vi "WhatDoNow.vi"(10 "Target":dbl(slide) scale=-3.14159..3.14159, 11 "Current":dbl(slide) scale=-3.14159..3.14159) -> (2 "Invert":bool, 3 "Output":dbl)   [LabVIEW 2013]
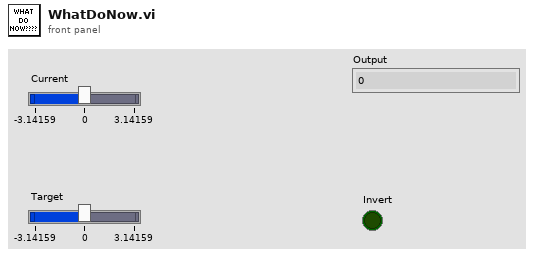
[diagram p1: front panel]
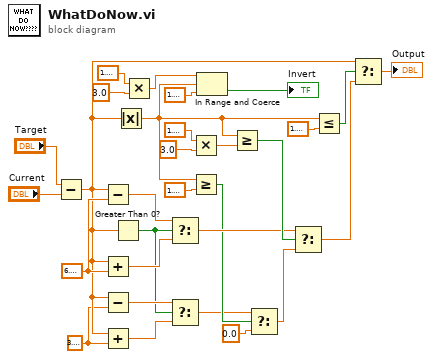
[diagram p0: block diagram]
diagram:
  w9 = 3.141592653589793
  w17 = 6.283185307179586
  n1 = Subtract(x="Target", y="Current") -> (x-y=w11:dbl)
  n2 = Subtract(x=w11, y=w17) -> (x-y=w19:dbl)
  n3 = Add(x=w11, y=w17) -> (x+y=w18:dbl)
  n4 = Subtract(x=w11, y=w9) -> (x-y=w10:dbl)
  n5 = Add(x=w11, y=w9) -> (x+y=w12:dbl)
  n6 = Greater Than 0?(x=w11) -> (x > 0?=w1:bool)
  n7 = Absolute Value(x=w11) -> (abs(x)=w6:dbl)
  n8 = Multiply(x=1.5707963267948966, y=3.0) -> (x*y=w2:dbl)
  n9 = Select(t=w19, s=w1, f=w18) -> (s? t:f=w20:dbl)
  n10 = Select(t=w10, s=w1, f=w12) -> (s? t:f=w13:dbl)
  n11 = Multiply(x=1.5707963267948966, y=3.0) -> (x*y=w25:dbl)
  n12 = Greater Or Equal?(x=w6, y=1.5707963267948966) -> (x >= y?=w15:bool)
  n13 = In Range and Coerce(upper limit=w2, x=w6, lower limit=1.5707963267948966) -> (In Range?=→"Invert":bool)  [unwired: 1 out]
  n14 = Greater Or Equal?(x=w6, y=w25) -> (x >= y?=w21:bool)
  n15 = Select(t=w13, s=w15, f=0.0) -> (s? t:f=w16:dbl)
  n16 = Select(t=w20, s=w21, f=w16) -> (s? t:f=w22:dbl)
  n17 = Less Or Equal?(x=w6, y=1.5707963267948966) -> (x <= y?=w27:bool)
  n18 = Select(t=w11, s=w27, f=w22) -> (s? t:f=→"Output":dbl)
